vi "Field Emission.vi"(10 "Velocity":dbl, 11 "Pelletron Volts":dbl) -> (3 "Field Emission":dbl)   [LabVIEW 2012]
panel:
  # "Field \nEmission=(2*pelletronvolts./v.^2*3e9*4*pi*8.854187817e-12).^3*(3/(4*pi*3200))^2;"
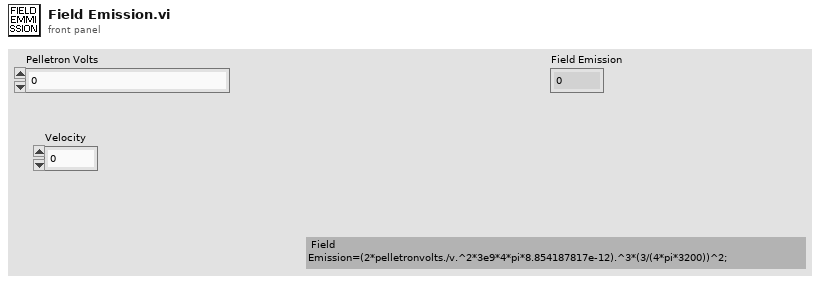
[diagram p1: front panel]
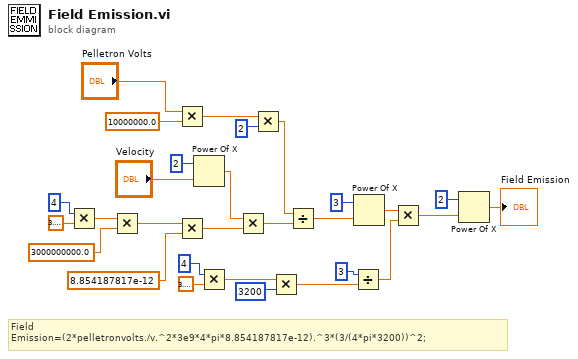
[diagram p0: block diagram]
diagram:
  # "Field \nEmission=(2*pelletronvolts./v.^2*3e9*4*pi*8.854187817e-12).^3*(3/(4*pi*3200))^2;"
  n1 = Multiply(x=4, y=3.141592653589793) -> (x*y=w23:dbl)
  n2 = Multiply(x=w23, y=3000000000.0) -> (x*y=w21:dbl)
  n3 = Multiply(x="Pelletron Volts", y=10000000.0) -> (x*y=w2:dbl)
  n4 = Multiply(x=w21, y=8.854187817e-12) -> (x*y=w18:dbl)
  n5 = Power Of X(1:"Velocity", 2:2 ("y")) -> (0:w19:dbl)
  n6 = Multiply(x=4 ("y"), y=3.141592653589793) -> (x*y=w6:dbl)
  n7 = Multiply(x=w19, y=w18) -> (x*y=w16:dbl)
  n8 = Multiply(x=w2, y=2) -> (x*y=w28:dbl)
  n9 = Multiply(x=w6, y=3200) -> (x*y=w4:dbl)
  n10 = Divide(x=w28, y=w16) -> (x/y=w15:dbl)
  n11 = Divide(x=3, y=w4) -> (x/y=w9:dbl)
  n12 = Power Of X(1:w15, 2:3) -> (0:w14:dbl)
  n13 = Multiply(x=w14, y=w9) -> (x*y=w13:dbl)
  n14 = Power Of X(1:w13, 2:2) -> (0:→"Field Emission":dbl)
